vi "New Dictionary (Wfm Data Refs).vi"(8 "error in (no error)":errorcluster, 11 "Wfm Data Refs":T1[](array[typedef])) -> (0 "error out":errorcluster, 3 "Dictionary out":refnum<class "Reference Dictionary.lvclass">)   [LabVIEW 2012, in "Waveform Data Logger Engine.lvlib" / "Reference Dictionary.lvclass"]
uses:
  Reference Dictionary.lvclass
  <vilib>/NI Veristand/Custom Device API/Waveform Data Reference.ctl
  Reference Dictionary.lvclass/Reference Dictionary.ctl
  <vilib>/NI VeriStand/Custom Device API/Custom Device API.lvlib
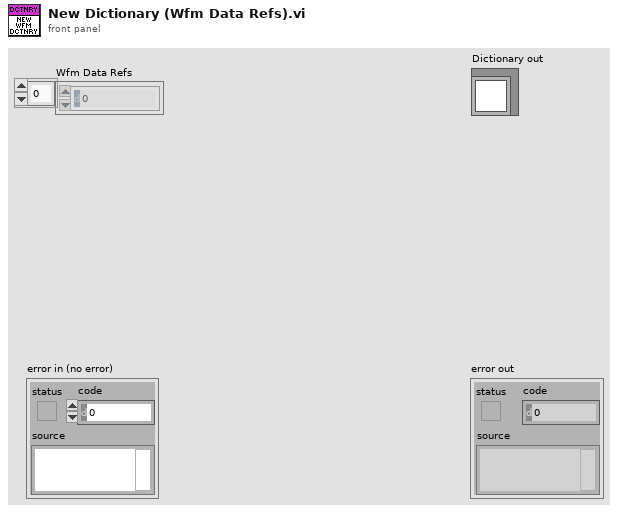
[diagram p1: front panel]
types:
  T1 = typedef "Custom Device API.lvlib/Waveform Data Reference.ctl" = i32
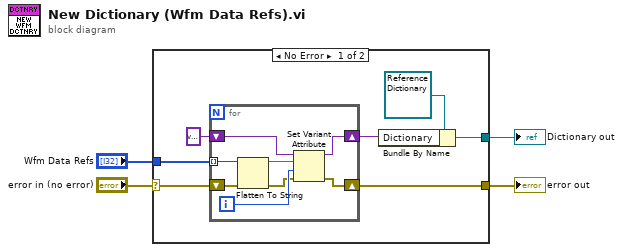
[diagram p0: block diagram]
diagram:
  n1 = case shown="No Error" "error in (no error)" {
    selector: "error in (no error)" -> [w10 w20]
    tunnel: [w9 w20] -> w3
    tunnel: [w11 _] -> w1
    tunnel: "Wfm Data Refs" -> [w8 _]
    frame No Error {
      n2 = for {
        shift-right: [w12] -> w7
        shift-left: variant ("Dictionary") -> [w15]
        shift-right: [w13] -> w9
        shift-left: w10 -> [w18]
        tunnel: w8 -> [w16] mode=indexing
        i -> [w19]
        n3 = Flatten To String(anything=w16, error in (no error)=w18) -> (data string=w14:string, error out=w17:errorcluster)  [unwired: 2 in, 1 out]
        n4 = Set Variant Attribute(Variant=w15, name=w14, value=w19, error in=w17) -> (Variant out=w12:variant, error out=w13:errorcluster)  [unwired: 1 out]
      }
      n5 = Bundle By Name(cluster=refnum<class "Reference Dictionary.lvclass"> refnum ("Dictionary out"), "Dictionary"=w7) -> (w11:refnum<class "Reference Dictionary.lvclass">)
    }
    frame Error {
    }
  }
  "error out" <- w3
  "Dictionary out" <- w1
